vi "GetFileVersionInfo_Main.vi"(8 "error in (no error)":errorcluster, 11 "Exe Path (Calling App)":path) -> (0 "error out":errorcluster, 1 "FileVersionInfo Out":T1, 2 "File Version Info":string, 3 "Path Out":path)   [LabVIEW 2015]
doc: "This VI can obtain information about an existing executable, such as its version, product name, and so on, or it can be called as a subVI from a VI that will be built into an executable to obtain information about that executable.\n\nTo obtain version information about an existing executable, enter a path to an executable into Exe Path and run the Vi.\n\nCall this VI as a subVI from a VI that you will build into an executable and leave the path input unwired to obtain the version information about the built executable."
panel:
  # "This VI can obtain information about an\nexisting executable, such as its\nversion, product name, and so on, or it\ncan be called as a subVI from a VI\nthat will be built into an executable to\nobtain information about that\nexecutable.\n\nTo obtain version information about an\nexisting executable, enter a path to an\nexecutable into Exe Path and run the Vi.\n\nCall this VI as a subVI from a VI that\nyou will build into an executable and\nleave the path input unwired to\nobtain the version information about\nthe built executable."
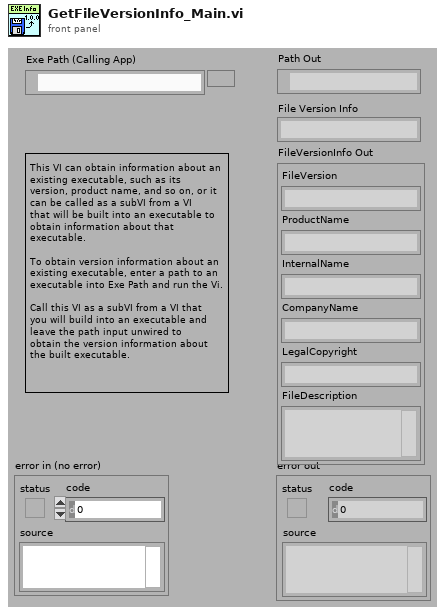
[diagram p1: front panel]
types:
  T1 = cluster{"FileVersion":string, "ProductName":string, "InternalName":string, "CompanyName":string, "LegalCopyright":string, "FileDescription":string}
  T2 = enum16{"CharacterArray", "FixedFileInfoCluster", "LanguageCode"}
  T3 = cluster{"[0]":string, "[1]":string, "[2]":string, "[3]":string, "[4]":string, "[5]":string}
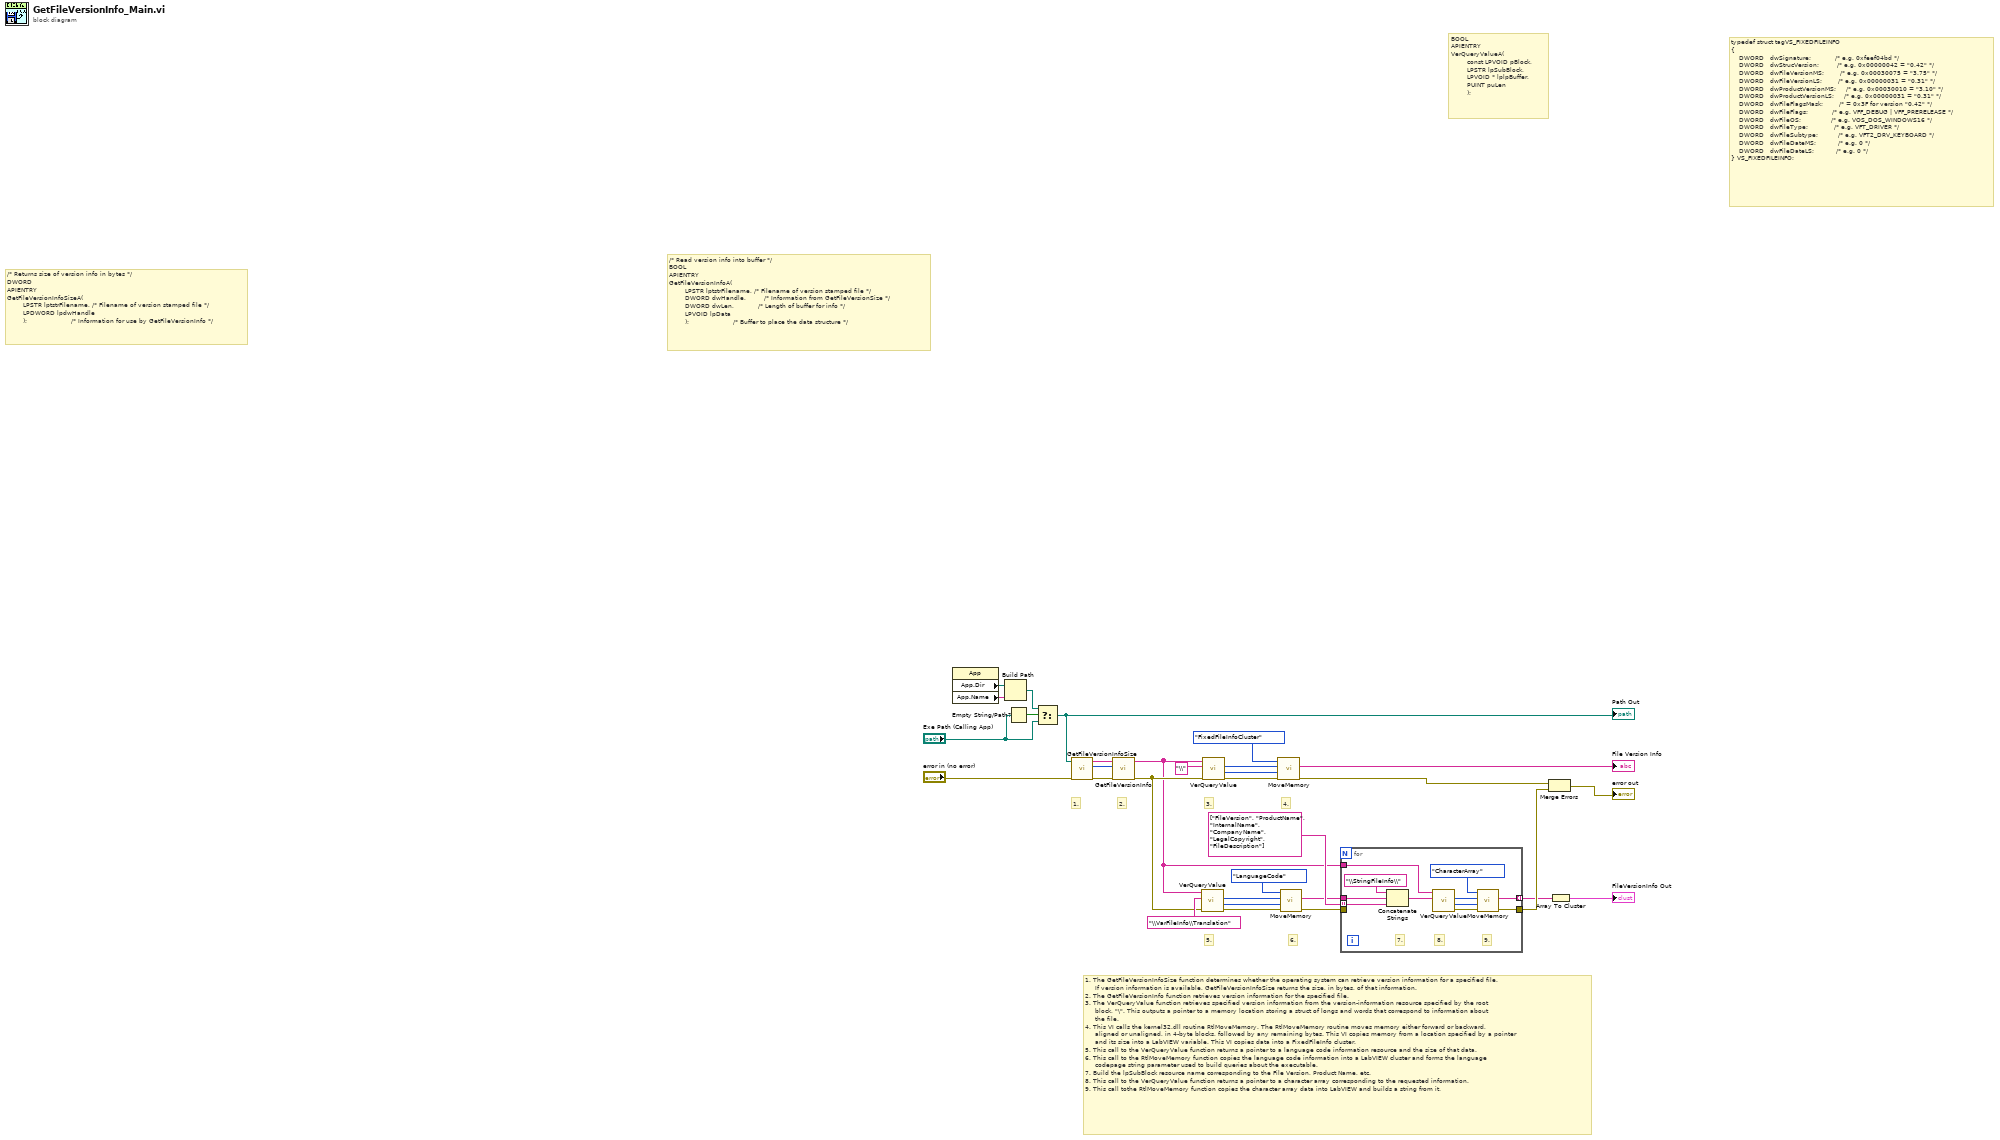
[diagram p0: block diagram]
diagram:
  # "6."
  # "4."
  # "5."
  # "3."
  # "2."
  # "1. The GetFileVersionInfoSize function determines whether the operating system can retrieve version information for a specified file.\n     If version information is available, GetFileVersionInfoSize returns the size, in bytes, of that information.\n2. The GetFileVersionInfo function retrieves version information for the specified file.\n3. The VerQueryValue function retrieves specified version information from the version-information resource specified by the root\n     block, \"\\\". This outputs a pointer to a memory location storing a struct of longs and words that correspond to information about\n     the file.\n4. This VI calls the kernel32.dll routine RtlMoveMemory. The RtlMoveMemory routine moves memory either forward or backward,\n     aligned or unaligned, in 4-byte blocks, followed by any remaining bytes. This VI copies memory from a location specified by a pointer\n     and its size into a LabVIEW variable. This VI copies data into a FixedFileInfo cluster. \n5. This call to the VerQueryValue function returns a pointer to a language code information resource and the size of that data.\n6. This call to the RtlMoveMemory function copies the language code information into a LabVIEW cluster and forms the language\n     codepage string parameter used to build queries about the executable.\n7. Build the lpSubBlock resource name corresponding to the File Version, Product Name, etc. \n8. This call to the VerQueryValue function returns a pointer to a character array corresponding to the requested information.\n9. This call tothe RtlMoveMemory function copies the character array data into LabVIEW and builds a string from it."
  # "1."
  # "/* Returns size of version info in bytes */\nDWORD\nAPIENTRY\nGetFileVersionInfoSizeA(\n        LPSTR lptstrFilename, /* Filename of version stamped file */\n        LPDWORD lpdwHandle\n        );                      /* Information for use by GetFileVersionInfo */"
  # "typedef struct tagVS_FIXEDFILEINFO\n{\n    DWORD   dwSignature;            /* e.g. 0xfeef04bd */\n    DWORD   dwStrucVersion;         /* e.g. 0x00000042 = \"0.42\" */\n    DWORD   dwFileVersionMS;        /* e.g. 0x00030075 = \"3.75\" */\n    DWORD   dwFileVersionLS;        /* e.g. 0x00000031 = \"0.31\" */\n    DWORD   dwProductVersionMS;     /* e.g. 0x00030010 = \"3.10\" */\n    DWORD   dwProductVersionLS;     /* e.g. 0x00000031 = \"0.31\" */\n    DWORD   dwFileFlagsMask;        /* = 0x3F for version \"0.42\" */\n    DWORD   dwFileFlags;            /* e.g. VFF_DEBUG | VFF_PRERELEASE */\n    DWORD   dwFileOS;               /* e.g. VOS_DOS_WINDOWS16 */\n    DWORD   dwFileType;             /* e.g. VFT_DRIVER */\n    DWORD   dwFileSubtype;          /* e.g. VFT2_DRV_KEYBOARD */\n    DWORD   dwFileDateMS;           /* e.g. 0 */\n    DWORD   dwFileDateLS;           /* e.g. 0 */\n} VS_FIXEDFILEINFO;"
  # "/* Read version info into buffer */\nBOOL\nAPIENTRY\nGetFileVersionInfoA(\n        LPSTR lptstrFilename, /* Filename of version stamped file */\n        DWORD dwHandle,         /* Information from GetFileVersionSize */\n        DWORD dwLen,            /* Length of buffer for info */\n        LPVOID lpData\n        );                      /* Buffer to place the data structure */"
  # "BOOL\nAPIENTRY\nVerQueryValueA(\n        const LPVOID pBlock,\n        LPSTR lpSubBlock,\n        LPVOID * lplpBuffer,\n        PUINT puLen\n        );"
  n1 = property class="App"() -> ("App.Dir"=w13:path, "App.Name"=w12:string)  [unwired: 2 in, 2 out]
  n2 = Build Path(base path=w13, name or relative path=w12) -> (appended path=w10:path)
  n3 = Empty String/Path?(string/path="Exe Path (Calling App)") -> (empty?=w11:bool)
  n4 = Select(t=w10, s=w11, f="Exe Path (Calling App)") -> (s? t:f=w8:path)
  "Path Out" <- w8
  n5 = call "GetFileVersionInfoSize.vi"("error in (no error)"="error in (no error)", "Path"=w8) -> ("error out"=w16:errorcluster, "Size"=w15:i32, "lptstrFilename"=w17:string)  [unwired: 7 in]
  n6 = call "GetFileVersionInfo.vi"("error in"=w16, "Size"=w15, "lptstrFilename"=w17) -> ("error out"=w19:errorcluster, "lpData"=w2:string)  [unwired: 7 in]
  n7 = call "VerQueryValue.vi"("error in (no error)"=w19, "lpSubBlock"="\\VarFileInfo\\Translation", "lpData"=w2) -> ("error out"=w20:errorcluster, "puLen"=w22:i32, "lplpBuffer"=w21:i32)  [unwired: 6 in]
  n8 = call "VerQueryValue.vi"("error in (no error)"=w19, "lpSubBlock"="\\", "lpData"=w2) -> ("error out"=w29:errorcluster, "puLen"=w26:i32, "lplpBuffer"=w27:i32)  [unwired: 6 in]
  n9 = call "MoveMemory.vi"("error in (no error)"=w29, "puLen"=w26, "lplpBuffer"=w27, "Datatype"=T2."FixedFileInfoCluster") -> ("error out"=w6:errorcluster, "data"=→"File Version Info":string)  [unwired: 6 in]
  n10 = call "MoveMemory.vi"("error in (no error)"=w20, "puLen"=w22, "lplpBuffer"=w21, "Datatype"=T2."LanguageCode") -> ("error out"=w18:errorcluster, "data"=w1:string)  [unwired: 6 in]
  n11 = for {
    tunnel: w2 -> [w39]
    tunnel: string[] ["FileVersion", "ProductName", "InternalName", "CompanyName", "LegalCopyright", "FileDescription"] -> [w41] mode=indexing
    tunnel: w18 -> [_]
    tunnel: [w34] -> w7
    tunnel: [w33] -> w4 mode=indexing
    tunnel: w1 -> [w32]
    # "7."
    # "9."
    # "8."
    n12 = Concatenate Strings("\\StringFileInfo\\" ("lpSubBlock"), w32, w41) -> (w40:string)
    n13 = call "VerQueryValue.vi"("lpSubBlock"=w40, "lpData"=w39) -> ("error out"=w37:errorcluster, "puLen"=w35:i32, "lplpBuffer"=w36:i32)  [unwired: 7 in]
    n14 = call "MoveMemory.vi"("error in (no error)"=w37, "puLen"=w35, "lplpBuffer"=w36, "Datatype"=T2."CharacterArray") -> ("error out"=w34:errorcluster, "data"=w33:string)  [unwired: 6 in]
  }
  n15 = Merge Errors(w6, w7) -> (→"error out":errorcluster)
  n16 = Array To Cluster(array=w4) -> (cluster=→"FileVersionInfo Out":T3)
